vi "20201104 pre003 position_theta measurement after bonding.vi"() -> ()   [LabVIEW 2016]
panel:
  out "X position":dbl[](array[numeric]) format="%#_8g"
  out "Yposition":dbl[](array[numeric]) format="%#_8g"
  out "Array":dbl[](array[numeric]) format="%#_8g"
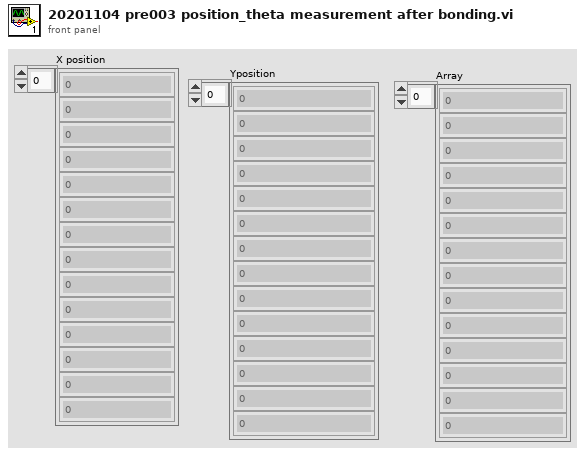
[diagram p1: front panel]
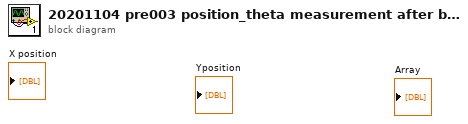
[diagram p0: block diagram]
diagram:
